vi "Launch Blower Actor.vi"(0 "Caller Actor in":refnum<class "Actor.lvclass">, 1 "Name":string, 2 "DedicatedEnQrs":refnum<queue>, 3 "Start Action (Open)":T2, 5 "Interlock Chain":refnum<class "Interlock Chain.lvclass">, 7 "SHV Aliases":refnum<k21>[](array[refnum]), 9 "Freezer":T1, 11 "error in (no error)":errorcluster, 12 "SHV":refnum<k21>[](array[refnum]), 14 "Stop Action (Close)":T2=enum."Close") -> (4 "Caller-To-Actor Enqueuer":refnum<class "Message Enqueuer.lvclass">, 15 "error out":errorcluster)   [LabVIEW 2015, in "cRIO-Carbondioxide.lvlib" / "CO2-Actor.lvlib" / "Blower.lvclass"]
uses:
  Blower.lvclass
  <vilib>/ActorFramework/Actor/Actor.lvclass
  Interlocks/Interlock Chain/Interlock Chain.lvclass
  <vilib>/ActorFramework/Message Enqueuer/Message Enqueuer.lvclass
  Valve/Action.ctl
  cRIO-CO2/Freezers Enumerator.ctl
  Controls/Dedicated Enqueuers.ctl
  CO2 Actor/CO2 Actor.lvclass
  Valve/Valve.lvclass/Valve.ctl
  Blower.lvclass/Blower.ctl
  Valve/Valve.lvclass
  cRIO-CO2/cRIO-CO2.lvclass
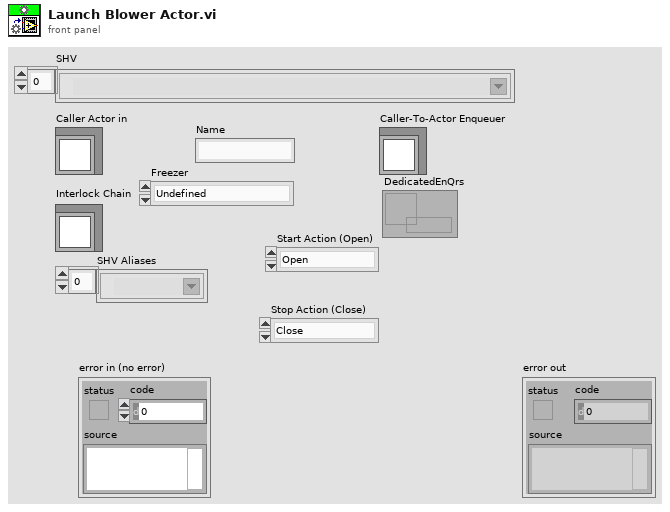
[diagram p1: front panel]
types:
  T1 = typedef "cRIO-Carbondioxide.lvlib/cRIO-CO2.lvlib/cRIO-CO2.lvclass/Freezers Enumerator.ctl" = enum16{"Undefined", "Syringe", "Cold Tank 1", "Cold Tank 2", "Cold Tank 3", "Cold Tank 4"}
  T2 = typedef "Action.ctl" = enum16{"Open", "Close", "None"}
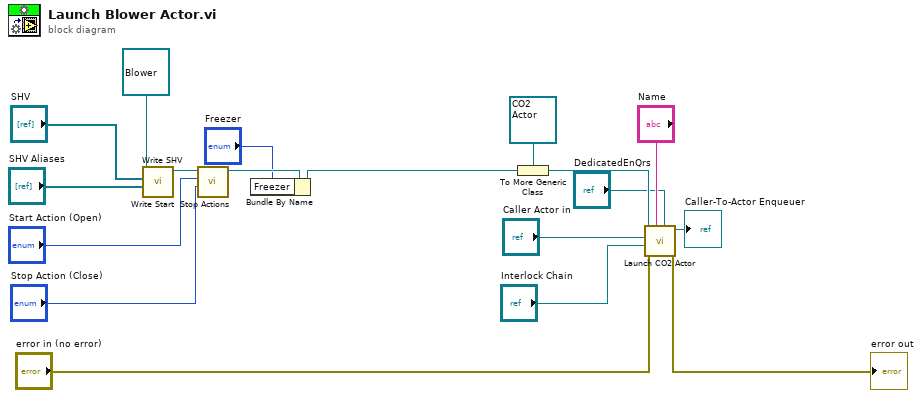
[diagram p0: block diagram]
diagram:
  n1 = call "Write SHV.vi"("SHV Aliases"="SHV Aliases", "SHV"="SHV", "Valve in"=refnum<class "Blower.lvclass"> refnum) -> ("Valve out"=w8:refnum<class "Blower.lvclass">)  [unwired: 8 in]
  n2 = call "Write Start  Stop Actions.vi"("Stop Action"="Stop Action (Close)", "Start Action"="Start Action (Open)", "Valve in"=w8) -> ("Valve out"=w5:refnum<class "Blower.lvclass">)  [unwired: 8 in]
  n3 = Bundle By Name(cluster=w5, "Freezer"="Freezer") -> (w1:refnum<class "Blower.lvclass">)
  n4 = To More Generic Class(target class=refnum<class "CO2 Actor.lvclass"> refnum ("CO2 Actor in"), reference=w1) -> (generic class reference=w12:refnum<class "CO2 Actor.lvclass">)
  n5 = call "Launch CO2 Actor.vi"("DedicatedEnQrs"="DedicatedEnQrs", "Name"="Name", "error in (no error)"="error in (no error)", "Interlock Chain"="Interlock Chain", "Caller Actor in"="Caller Actor in", "CO2 Actor in"=w12) -> ("error out"=→"error out":errorcluster, "Caller-To-Actor Enqueuer"=→"Caller-To-Actor Enqueuer":refnum<class "Message Enqueuer.lvclass">)  [unwired: 4 in]
